vi "MILStateFeedbackControllerY.vi"(0 "Ac":dbl[](array[numeric])=[0.0, 0.0, 0.0, 0.0], 1 "DispX":dbl, 2 "P1X":dbl, 3 "DispY":dbl, 5 "Bc":dbl[](array[numeric])=[0.0, 0.0, 0.0, 0.0], 7 "Cc":dbl[](array[numeric])=[1.0, 0.0], 9 "Dc":dbl[](array[numeric])=[0.0, 0.0], 12 "ForceX":dbl, 13 "P2X":dbl, 14 "ForceY":dbl) -> (4 "ValveCMDX":dbl, 6 "ValveCMDY":dbl, 8 "StateY":dbl[](array[numeric]))   [LabVIEW 2020]
uses:
  <vilib>/Analysis/NI_AALBase.lvlib
  <vilib>/Analysis/NI_AALBLAS.lvlib
  <vilib>/Analysis/baseanly.llb/A x Vector.vi
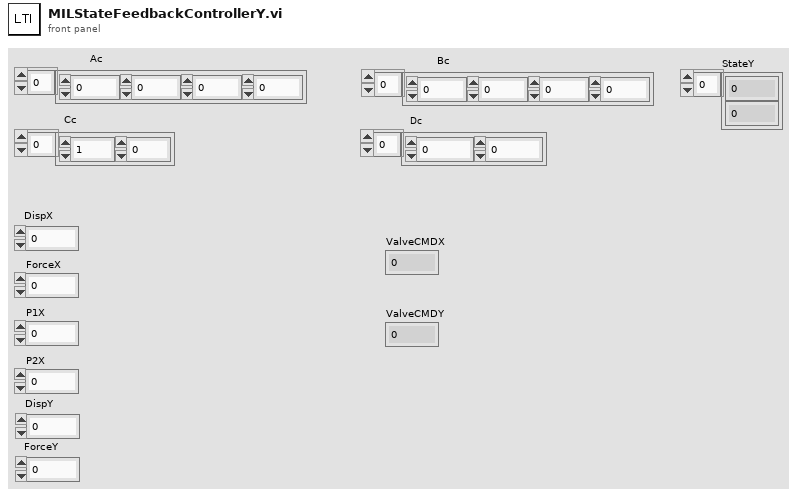
[diagram p1: front panel]
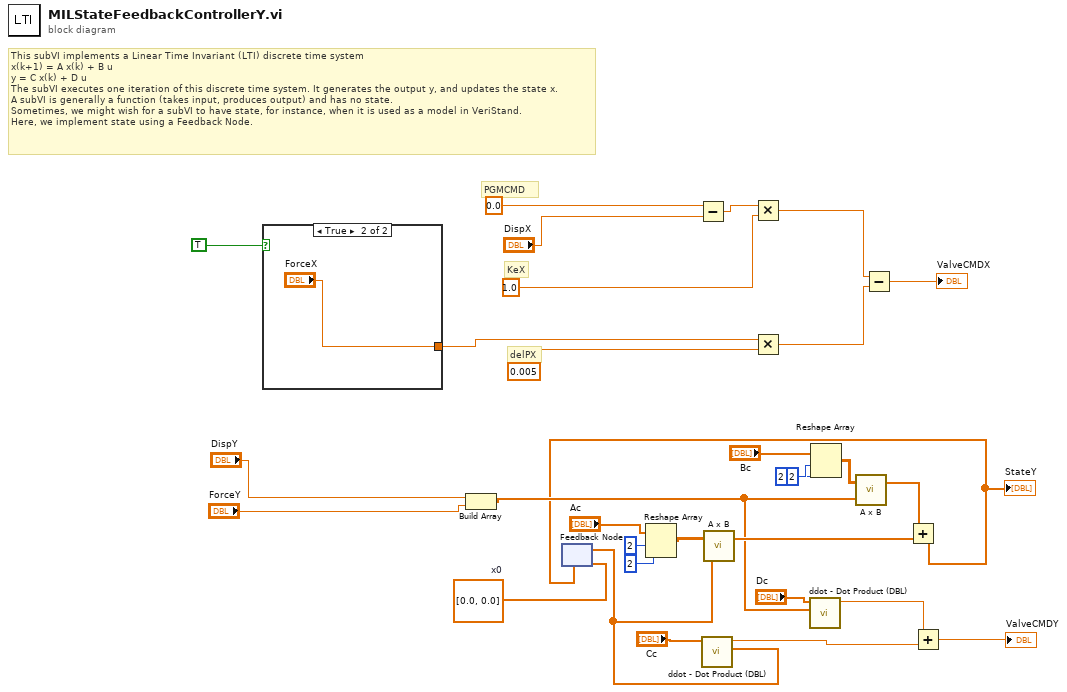
[diagram p0: block diagram]
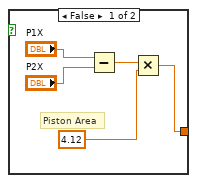
[diagram p2: hidden frame]
diagram:
  w31 = dbl[] [0.0, 0.0]  # x0
  # "PGMCMD"
  # "delPX"
  # "KeX"
  # "This subVI implements a Linear Time Invariant (LTI) discrete time system\nx(k+1) = A x(k) + B u\ny = C x(k) + D u\nThe subVI executes one iteration of this discrete time system. It generates the output y, and updates the state x.\nA subVI is generally a function (takes input, produces output) and has no state.\nSometimes, we might wish for a subVI to have state, for instance, when it is used as a model in VeriStand.\nHere, we implement state using a Feedback Node."
  n1 = case shown="True" TRUE {
    tunnel: [w32 "ForceX"] -> w1
    frame False {
      # "Piston Area"
      n2 = Subtract(x="P1X", y="P2X") -> (x-y=w36:dbl)
      n3 = Multiply(x=w36, y=4.12) -> (x*y=w32:dbl)
    }
    frame True {
    }
  }
  n4 = Build Array("DispY", "ForceY") -> (w25:dbl[])
  n5 = feedback #1(w31) -> (w29:dbl[])
  n6 = Reshape Array("Ac", 2 ("dimension size"), 2 ("dimension size")) -> (w22:dbl[][])
  n7 = Subtract(x=0.0 ("PGMCMDY"), y="DispX") -> (x-y=w12:dbl)
  n8 = call <vilib>:"ddot - Dot Product (DBL).vi"("y"=w29, "x"="Cc") -> ("ddot"=w28:dbl)  [unwired: 8 in, 1 out]
  n9 = call-poly <vilib>:"A x B.vi"("Vector"=w29, "A"=w22) -> ("A x Vector"=w30:dbl[])  [unwired: 1 out]
  n10 = Multiply(x=w12, y=1.0 ("KeY")) -> (x*y=w9:dbl)
  n11 = Multiply(x=w1, y=0.005 ("delPY")) -> (x*y=w8:dbl)
  n12 = call <vilib>:"ddot - Dot Product (DBL).vi"("y"=w25, "x"="Dc") -> ("ddot"=w26:dbl)  [unwired: 8 in, 1 out]
  n13 = Reshape Array("Bc", 2 ("dimension size"), 2 ("dimension size")) -> (w19:dbl[][])
  n14 = call-poly <vilib>:"A x B.vi"("Vector"=w25, "A"=w19) -> ("A x Vector"=w27:dbl[])  [unwired: 1 out]
  n15 = Subtract(x=w9, y=w8) -> (x-y=→"ValveCMDX":dbl)
  n16 = Add ("Add.vi")(x=w27, y=w30) -> (x+y=w18:dbl[])
  "StateY" <- w18
  n17 = feedback-in #1(w18) -> ()
  n18 = Add(x=w26, y=w28) -> (x+y=→"ValveCMDY":dbl)
